vi "Set Telemetry Config.vi"(8 "error in (no error)":errorcluster, 10 "Telemtry Config":T1, 11 "Node Config in":refnum<class "Node Config.lvclass">) -> (0 "error out":errorcluster, 3 "Node Config out":refnum<class "Node Config.lvclass">)   [LabVIEW 2020, in "VectoConfig.lvlib" / "Node Config.lvclass"]
uses:
  Node Config.lvclass
  Node Config.lvclass/Node Config.ctl
  VectoConfig/Telemetry Routing.ctl
  VectoConfig/VectoConfig.lvlib
  VectoConfig/Endpoint.ctl
  VectoConfig/Telemetry Config.ctl
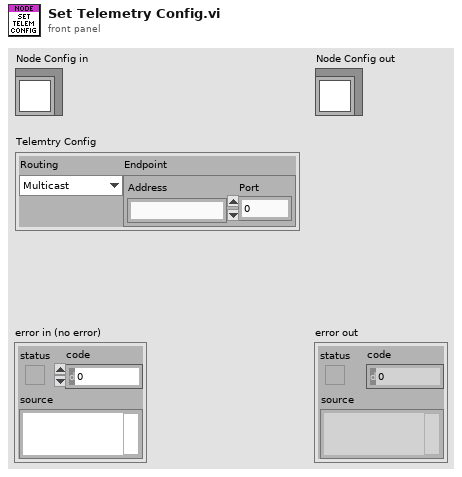
[diagram p1: front panel]
types:
  T1 = typedef "VectoConfig.lvlib/Telemetry Config.ctl" = cluster{"Routing":T2, "Endpoint":T3}
  T2 = typedef "VectoConfig.lvlib/Telemetry Routing.ctl" = enum16{"Multicast", "Unicast"}
  T3 = typedef "VectoConfig.lvlib/Endpoint.ctl" = cluster{"Address":string, "Port":u16}
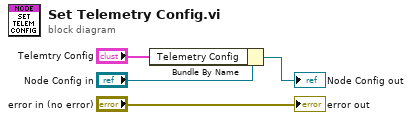
[diagram p0: block diagram]
diagram:
  n1 = Bundle By Name(cluster="Node Config in", "Telemetry Config"="Telemtry Config") -> (→"Node Config out":refnum<class "Node Config.lvclass">)
  "error out" <- "error in (no error)"
